vi "DS345.set delay gate.vi"(0 "i ref in":refnum<vi>, 1 "sampleFrequency [Hz]":dbl min=0.0 max=1500.0 step=1.0 format="%.3f", 2 "delay [us]":dbl min=0.0 max=1500.0 step=1.0 format="%.3f", 4 "gate [us]":dbl min=0.0 max=1500.0 step=1.0 format="%.3f", 5 "error in (no error)":errorcluster) -> (14 "i ref out":refnum<vi>, 19 "error out":errorcluster)   [LabVIEW 2014, in "DS345.lvlib"]
doc: "sets the delay and gate values for a DS345. By calling this method, the DS345 can be used as a delay gate generator that is externally triggered."
uses:
  DS345.lvlib
  CSCore/CSSystem/CoreLib/CoreLib.lvlib
  CSCore/CSSystem/CoreDefs/CoreDefs.error_type.ctl
  CSCore/CSApplicationBaseClasses/AFGBase/AFGBase.lvlib
  CSCore/CSApplicationBaseClasses/AFGBase/AFGBase.waveformType.ctl
  CSlibraries/UtilityLib/UtilityLib.valueStatus.ctl
  CSlibraries/UtilityLib/UtilityLib.lvlib
  CSCore/CSApplicationBaseClasses/DeviceBase/DeviceBase.lvlib
  CSCore/CSApplicationBaseClasses/DeviceBase/DeviceBase.deviceState.ctl
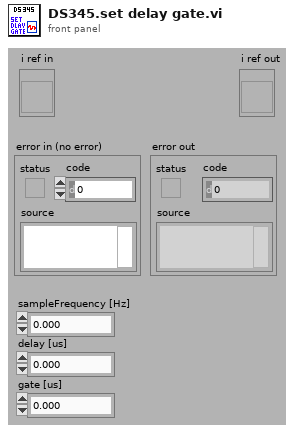
[diagram p1: front panel]
types:
  T1 = typedef "AFGBase.lvlib/AFGBase.waveformType.ctl" = enum16{"sine", "square", "ramp", "pulse", "noise", "DC", "arbitrary", "triangle", "ramp_up", "ramp_down", "amplitude modulation"}
  T2 = typedef "UtilityLib.lvlib/UtilityLib.valueStatus.ctl" = enum16{"no info available", "stand by/off", "on", "warning", "alarm/malfunction", "not implemented", "user action required", "important information", "system default", "control default", "indicator default", "button default"}
  T3 = typedef "CoreDefs.error_type.ctl" = enum16{"no error", "can't load process", "can't unload process", "process does not exist", "can't install process", "can't remove process", "unknown function", "time out", "can't execute function", "duplicate queue name", "super not found", "caller queue invalid", "can't ping process", "unknown error", "VISA Error", "VISA timeout", "GPIB timeout", "GPIB error", "communication error", "data type mismatch", "can't read data from OPC server", "can't write data to OPC server", "OET error", "function not implemented", "process already exists", "invalid Shared Variable name", "error writing Shared Variable", "error reading Shared Variable", "invalid client name", "corrupt database", "unknown class", "call not authorized", "parameter out of range", "OET timeout: can't get data to modify", "invalid queue name", "requested operation incompatible with current state", "event undefined", "event disabled", "state undefined", "caller is not a friend", "EventBuilder: bad eventID", "EventBuilder: no DAQ devices", "a thread must not stop itself", "UNUSED ELEMENT4", "DiscArchiver: eventData incomplete", "DiscArchiver: eventData does not belong to run", "DiscArchiver: can't open file", "DiscArchiver: can't write to file", "DiscArchiver: available disc space low", "can't acquire semaphore", "error reading data from database", "notifier object is not existing", "can't register process", "can't unregister process", "illegal event type", "object disabled", "object already exists", "can't change state", "Instrument not found", "no connection to remote node", "invalid reference", "N/A", "UNUSED ELEMENT 1", "element not found", "illegal TCP/IP connection detected", "object does not exist", "invalid access ID", "unknown CS system", "invalid privilige", "unsupported data type", "unsupported server type", "IO server already exists", "Shared Variable already exists"}
  T4 = typedef "DeviceBase.lvlib/DeviceBase.deviceState.ctl" = i16
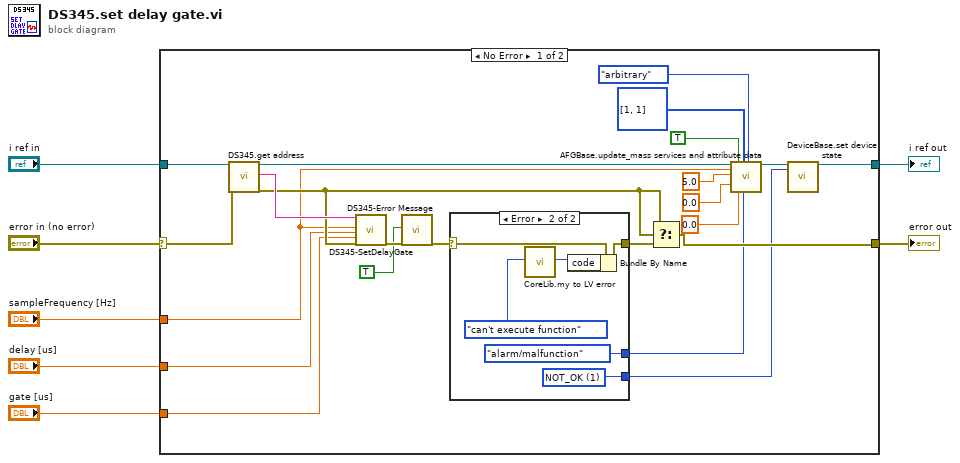
[diagram p0: block diagram]
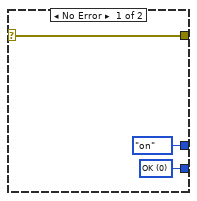
[diagram p2: hidden frame]
diagram:
  n1 = case shown="No Error" "error in (no error)" {
    selector: "error in (no error)" -> [w21 w40]
    tunnel: [w20 w40] -> w7
    tunnel: "i ref in" -> [w29 w41]
    tunnel: "sampleFrequency [Hz]" -> [w18 _]
    tunnel: "delay [us]" -> [w27 _]
    tunnel: "gate [us]" -> [w26 _]
    tunnel: [w9 w41] -> w2
    frame No Error {
      n2 = call "DS345.get address.vi"("i ref in"=w29, "error in (no error)"=w21) -> ("i ref out"=w19:refnum<vi>, "address"=w30:string, "error out"=w28:errorcluster)  [unwired: 15 in]
      n3 = call "DS345-SetDelayGate.vi"("address string"=w30, "sampleFrequency [Hz]"=w18, "delay [us]"=w27, "pulseLength [us["=w26, "error in (no error)"=w28) -> ("error out"=w25:errorcluster)  [unwired: 13 in, 1 out]
      n4 = call "DS345-Error Message.vi"("addMessageToSource"=TRUE ("add message to source"), "error in (no error)"=w25) -> ("error out"=w24:errorcluster)  [unwired: 14 in, 3 out]
      n5 = case shown="Error" w24 {
        selector: w24 -> [w33 w39]
        tunnel: [w33 w38] -> w22
        tunnel: [UtilityLib.valueStatus."on" ("valueStatus") UtilityLib.valueStatus."alarm/malfunction" ("valueStatus")] -> w11
        tunnel: [w31 w34] -> w8
        frame No Error {
          w31 = T4 0 items=["ERROR"=-1, "OK"=0, "NOT_OK"=1] ("deviceState")
        }
        frame Error {
          w34 = T4 1 items=["ERROR"=-1, "OK"=0, "NOT_OK"=1] ("deviceState")
          n6 = call "CoreLib.my to LV error.vi"("ErrorTypes"=CoreDefs.error_type."can't execute function") -> ("LV error code"=w37:i32)  [unwired: 17 in, 1 out]
          n7 = Bundle By Name(cluster=w39, "code"=w37) -> (w38:errorcluster)
        }
      }
      n8 = Select(t=w28, s=w28, f=w22) -> (s? t:f=w20:errorcluster)
      n9 = call "AFGBase.update_mass services and attribute data.vi"("i ref in"=w19, "frequency"=w18, "amplitude"=5.0, "phase"=0.0, "enableOutput"=TRUE, "DCOffset"=0.0, "trigger"=i16[] [1, 1], "valueStatus"=w11, "waveformType"=AFGBase.waveformType."arbitrary") -> ("i ref out"=w10:refnum<vi>)  [unwired: 8 in, 2 out]
      n10 = call "DeviceBase.set device state.vi"("i ref in"=w10, "deviceState"=w8) -> ("i ref out"=w9:refnum<vi>)  [unwired: 15 in, 2 out]
    }
    frame Error {
    }
  }
  "error out" <- w7
  "i ref out" <- w2
